vi "Create Channel Task Manual.vi"(8 "error in":errorcluster, 9 "Waveform Generation":T1(array[cluster]), 10 "SQL query":string="SELECT max(MaximumVoltage),max(MinimumVoltage), max(TerminalConfiguration),max(SampleRate) FROM ltt.daq_configuration \nWhere ChannelType='Analog_Output' and Enabled=1;", 11 "NI Analog Output in":refnum<class "NI Analog Output.lvclass">) -> (0 "error out":errorcluster, 3 "NI Analog Output out":refnum<class "NI Analog Output.lvclass">)   [LabVIEW 2023, in "HardwareAbstractionLayer_LVOOP.lvlib" / "NI Analog Output.lvclass"]
doc: "This VI Analog Output Physical Channel Based DAQmx Create Channel"
uses:
  NI Analog Output.lvclass
  NI Analog Output.lvclass/NI Analog Output.ctl
  <vilib>/DAQmx/create/channels.llb/DAQmx Create Channel (AO-Voltage-Basic).vi
  <vilib>/DAQmx/configure/timing.llb/DAQmx Timing (Sample Clock).vi
  Database/Database.lvclass
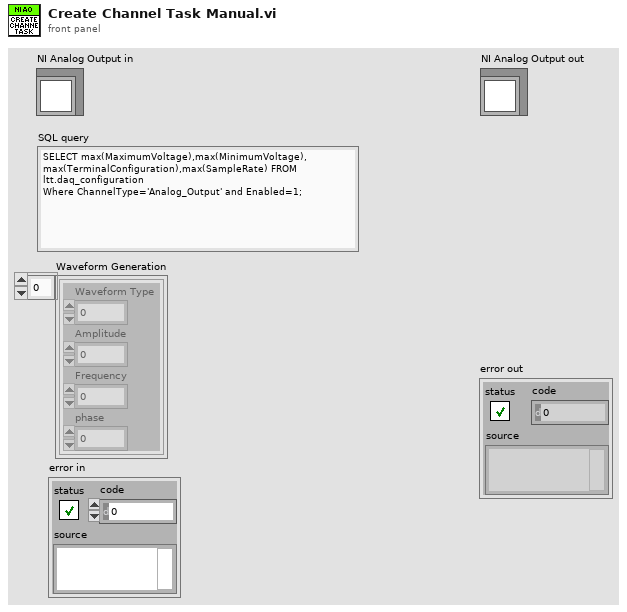
[diagram p1: front panel]
types:
  T1 = cluster{"Waveform Type":u16, "Amplitude":dbl, "Frequency":dbl, "phase":dbl}[]
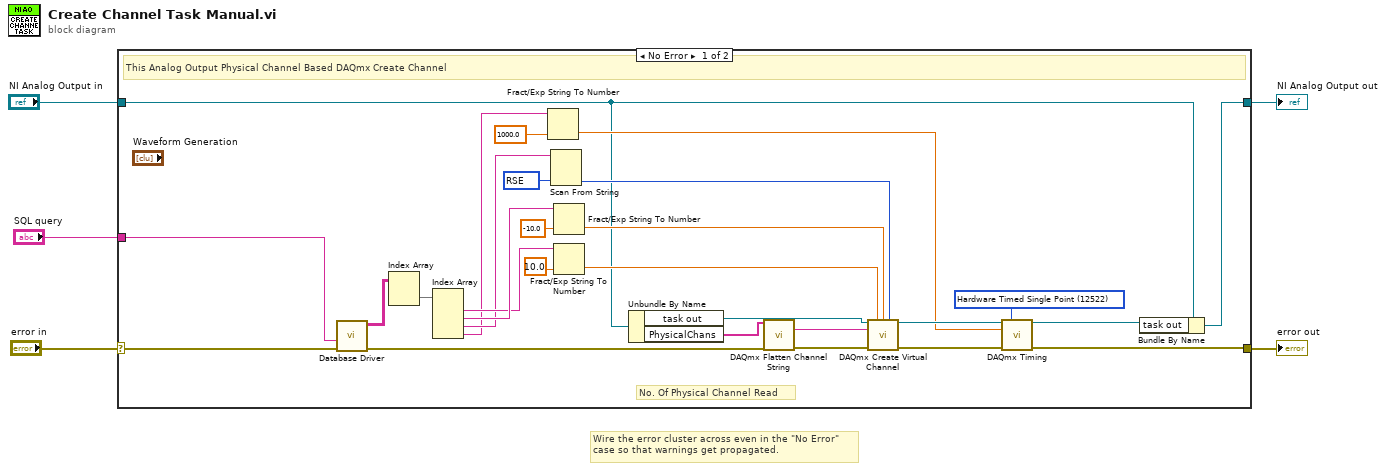
[diagram p0: block diagram]
diagram:
  # "Wire the error cluster across even in the \"No Error\"\ncase so that warnings get propagated."
  n1 = case shown="No Error" "error in" {
    selector: "error in" -> [w9 w35]
    tunnel: [w7 w35] -> w4
    tunnel: [w12 w34] -> w2
    tunnel: "NI Analog Output in" -> [w11 w34]
    tunnel: "SQL query" -> [w6 _]
    frame No Error {
      w14 = 12522 items=["Finite Samples"=10178, "Continuous Samples"=10123, "Hardware Timed Single Point"=12522] ("sample mode")
      w30 = 10083 items=["Default"=-1, "RSE"=10083, "NRSE"=10078, "Differential"=10106, "Pseudodifferential"=12529] ("input terminal configuration")
      # "No. Of Physical Channel Read"
      # "This Analog Output Physical Channel Based DAQmx Create Channel"
      n2 = call "Database Driver.vi"("error in"=w9, "SQL query"=w6) -> ("error out"=w8:errorcluster, "data"=w10:string[][])  [unwired: 6 in, 2 out]
      n3 = Index Array(array=w10) -> (element=w31:string[])  [unwired: 2 in]
      n4 = Index Array(array=w31) -> (element #1=w32:string, element #2=w33:string, element #3=w24:string, element #4=w16:string)  [unwired: 4 in]
      n5 = Fract/Exp String To Number(string=w16, default (0 dbl)=1000.0 ("rate")) -> (number=w15:dbl)  [unwired: 2 in, 1 out]
      n6 = Scan From String(input string=w24, default 1=w30) -> (output 1=w25:i32)  [unwired: 3 in, 3 out]
      n7 = Fract/Exp String To Number(string=w33, default (0 dbl)=-10.0 ("maximum value")) -> (number=w26:dbl)  [unwired: 2 in, 1 out]
      n8 = Fract/Exp String To Number(string=w32, default (0 dbl)=10.0 ("maximum value")) -> (number=w27:dbl)  [unwired: 2 in, 1 out]
      n9 = Unbundle By Name(w11) -> ("task out"=w20:refnum<k21>, "PhysicalChans"=w22:tag[])
      n10 = call <vilib>:"DAQmx Flatten Channel String.vi"("names in"=w22, "error in"=w8) -> ("names out"=w21:string, "error out"=w23:errorcluster)  [unwired: 12 in]
      n11 = call-poly <vilib>:"DAQmx Create Virtual Channel.vi"("task in"=w20, "maximum value"=w27, "minimum value"=w26, "output terminal configuration"=w25, "physical channels"=w21, "error in"=w23) -> ("task out"=w18:refnum<k21>, "error out"=w19:errorcluster)  [unwired: 8 in]
      n12 = call-poly <vilib>:"DAQmx Timing.vi"("task/channels in"=w18, "sample mode"=w14, "rate"=w15, "error in"=w19) -> ("task out"=w13:refnum<k21>, "error out"=w7:errorcluster)  [unwired: 10 in]
      n13 = Bundle By Name(cluster=w11, "task out"=w13) -> (w12:refnum<class "NI Analog Output.lvclass">)
    }
    frame Error {
    }
  }
  "error out" <- w4
  "NI Analog Output out" <- w2
